vi "Find Msgs.vi"(11 "TEMPLATE Actor in":refnum<class "{{Name}}Actor.lvclass">) -> (2 "Msgs":T1)   [LabVIEW 2020, in "_Template.lvlib" / "Templates.lvlib" / "{{Name}}Actor.lvlib" / "{{Name}}Actor.lvclass"]
uses:
  {{Name}}Actor.lvclass
  {{Name}}Actor.lvclass/{{Name}}Actor.ctl
  C:/jettl-harness/repos/jettl/src/jettl Tools/_Template/Templates/{{Name}}Actor/TEMPLATE Actor/{{Name}}Actor.lvclass
  C:/jettl-harness/repos/jettl/src/jettl/jettl/Actor/Actor.lvclass
  jettl/jettl/jettl.lvlib
  jettl/jettl/Message/Message.lvclass
  jettl/jettl/MessageSet.ctl
panel:
  # "This front panel should not be manipulated."
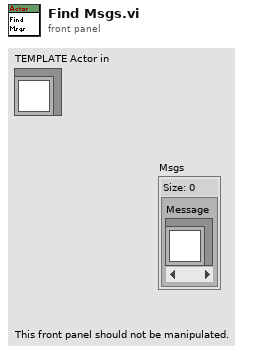
[diagram p1: front panel]
types:
  T1 = typedef "jettl.lvlib/MessageSet.ctl" = set{refnum<class "Message.lvclass">}
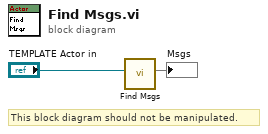
[diagram p0: block diagram]
diagram:
  # "This block diagram should not be manipulated."
  n1 = call "Find Msgs.vi"("X Actor.lvclass"="TEMPLATE Actor in") -> ("Msgs"=→"Msgs":T1)  [unwired: 10 in]
